vi "Video State.vi"() -> ()   [LabVIEW 2014]
panel:
  in  "Video Mode Control":enum16{"HatControl", "JoystickControl"}(ring)
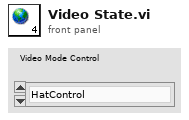
[diagram p1: front panel]
diagram:
